vi "digital_pulse.vi"() -> ()   [LabVIEW 2014]
doc: "Digital Pulse\nProgramma n impulsi sul DIO0 di polarita, durata e intervallo programmabili\n\nADL & FM 2011"
uses:
  <vilib>/DAQmx/write.llb/DAQmx Write (Digital Bool 1Line 1Point).vi
  <vilib>/DAQmx/create/channels.llb/DAQmx Create Channel (DO-Digital Output).vi
  <vilib>/DAQmx/miscellaneous.llb/DAQmx Fill In Error Info.vi
panel:
  in  "Numero impulsi":u8=2
  in  "Ritardo impulso (ms)":u32=10
  in  "Durata impulso (ms)":u32=10
  in  "Polarita impulso":bool=TRUE caption="ON\nOFF"
  # "Utilizzare il canale CB52 (linea digitale 0)"
  # "VERO"
  # "FALSO"
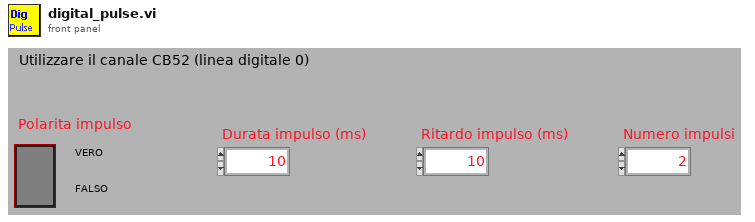
[diagram p1: front panel]
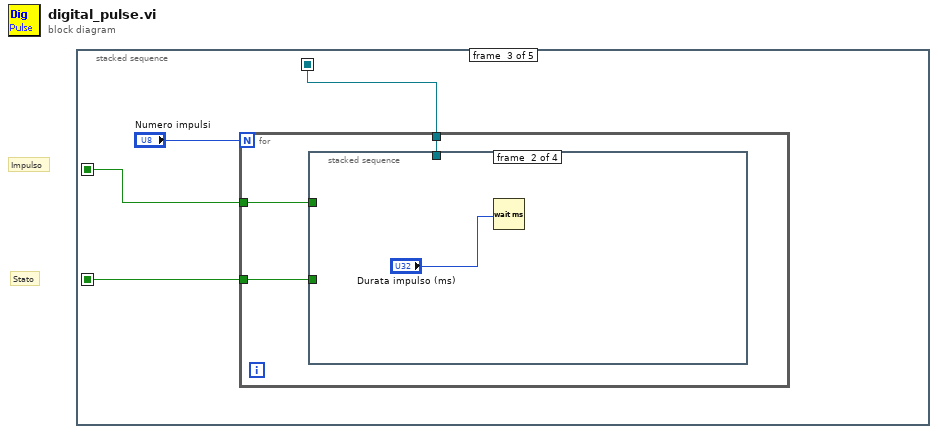
[diagram p0: block diagram]
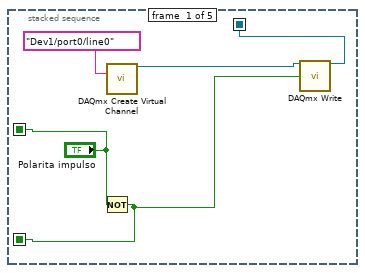
[diagram p2: hidden frame]
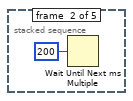
[diagram p3: hidden frame]
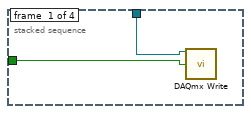
[diagram p4: hidden frame]
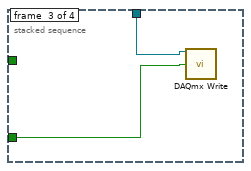
[diagram p5: hidden frame]
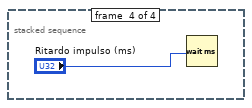
[diagram p6: hidden frame]
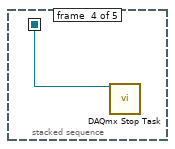
[diagram p7: hidden frame]
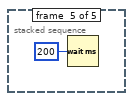
[diagram p8: hidden frame]
diagram:
  # "Stato"
  # "Impulso"
  n1 = stacked-sequence {
    seq-local: [w3 _ _ _ _] -> [_ _ w9 w20 _]
    seq-local: ["Polarita impulso" _ _ _ _] -> [_ _ w8 _ _]
    seq-local: [w1 _ _ _ _] -> [_ _ w7 _ _]
    frame #0 {
      n2 = Not(x="Polarita impulso") -> (.not. x?=w1:bool)
      n3 = call-poly <vilib>:"DAQmx Create Virtual Channel.vi"("lines"=tag "Dev1/port0/line0" ("Scelta linee")) -> ("task out"=w4:refnum<k21>)  [unwired: 4 in, 10 out]
      n4 = call-poly <vilib>:"DAQmx Write.vi"("task/channels in"=w4, "data"=w1) -> ("task out"=w3:refnum<k21>)  [unwired: 2 in, 11 out]
    }
    frame #1 {
      n5 = Wait Until Next ms Multiple(millisecond multiple=u32 200) -> ()  [unwired: 1 out]
    }
    frame #2 {
      n6 = for {
        N: "Numero impulsi" -> [_]
        tunnel: w9 -> [w13]
        tunnel: w8 -> [w12]
        tunnel: w7 -> [w11]
        n7 = stacked-sequence {
          tunnel: w13 -> [w15 _ w18 _]
          tunnel: w12 -> [w14 _ _ _]
          tunnel: w11 -> [_ _ w17 _]
          frame #0 {
            n8 = call-poly <vilib>:"DAQmx Write.vi"("task/channels in"=w15, "data"=w14) -> ()  [unwired: 2 in, 12 out]
          }
          frame #1 {
            n9 = Wait (ms)(milliseconds to wait="Durata impulso (ms)") -> ()  [unwired: 1 out]
          }
          frame #2 {
            n10 = call-poly <vilib>:"DAQmx Write.vi"("task/channels in"=w18, "data"=w17) -> ()  [unwired: 2 in, 12 out]
          }
          frame #3 {
            n11 = Wait (ms)(milliseconds to wait="Ritardo impulso (ms)") -> ()  [unwired: 1 out]
          }
        }
      }
    }
    frame #3 {
      n12 = call <vilib>:"DAQmx Stop Task.vi"("task/channels in"=w20) -> ()  [unwired: 1 in, 14 out]
    }
    frame #4 {
      n13 = Wait (ms)(milliseconds to wait=u32 200 ("millisecond multiple")) -> ()  [unwired: 1 out]
    }
  }
